vi "Stop Print Screw.vi"(8 "error in (no error)":errorcluster, 11 "Feeder Actor.lvlib:Screw.lvclass":refnum<class "Screw.lvclass">) -> (0 "error out":errorcluster, 3 "Feeder Actor.lvlib:Screw.lvclass 2":refnum<class "Screw.lvclass">)   [LabVIEW 2018]
uses:
  Screw.lvclass
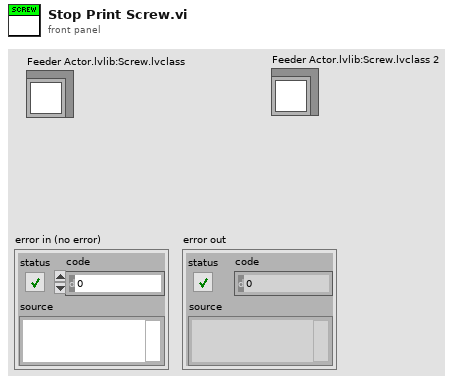
[diagram p1: front panel]
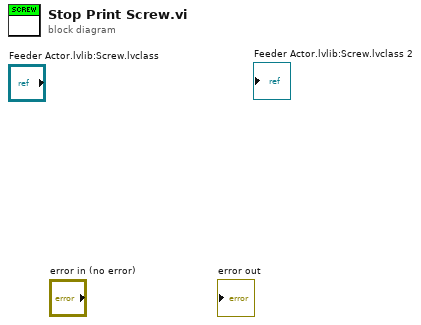
[diagram p0: block diagram]
diagram:
